vi "ExportDSAdata.vi"(8 "error in (no error)":errorcluster, 10 "Export Folder Path":path, 11 "Bode Plots":T1) -> (0 "error out":errorcluster)   [LabVIEW 2020, in "DynamicSignalAnalyzer.lvlib"]
doc: "Export DSA data to file"
uses:
  TypeDefs/BodePlot.ctl
  <vilib>/Utility/file.llb/Write Delimited Spreadsheet (DBL).vi
  DynamicSignalAnalyzer.lvlib
panel:
  in  "Pause Charts":bool
  # "For instructions on how to use the JKI State Machine Objects, examples and video tutorials, visit:\nhttp://jki.net/state-machine-objects/\n\nJKI State Machine Objects™\nhttp://jki.net/state-machine-objects/\nCopyright (C) 2005-2015, JKI <info@jki.net>\nALL RIGHTS RESERVED"
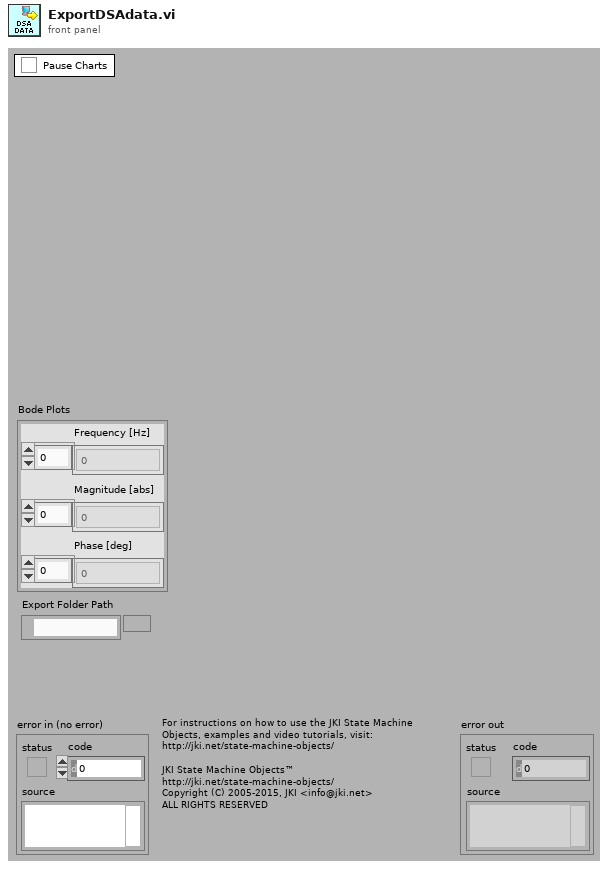
[diagram p1: front panel]
types:
  T1 = typedef "DynamicSignalAnalyzer.lvlib/BodePlot.ctl" = cluster{"Frequency [Hz]":dbl[], "Magnitude [abs]":dbl[], "Phase [deg]":dbl[]}
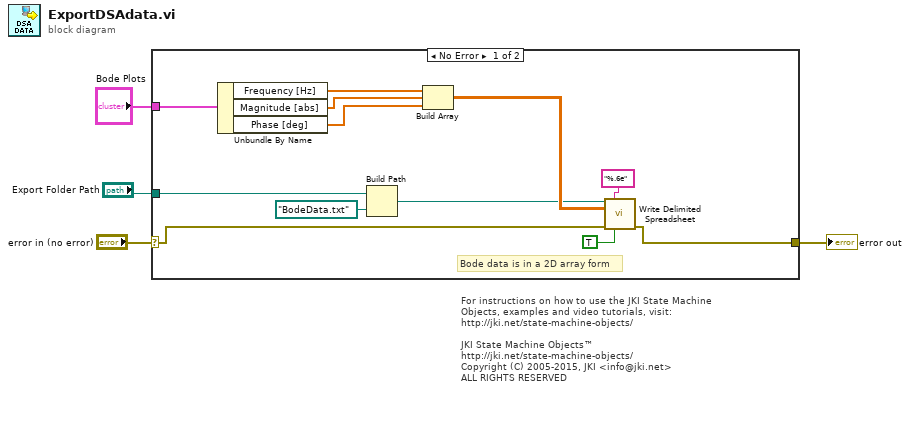
[diagram p0: block diagram]
diagram:
  # "For instructions on how to use the JKI State Machine Objects, examples and video tutorials, visit:\nhttp://jki.net/state-machine-objects/\n\nJKI State Machine Objects™\nhttp://jki.net/state-machine-objects/\nCopyright (C) 2005-2015, JKI <info@jki.net>\nALL RIGHTS RESERVED"
  n1 = case shown="No Error" "error in (no error)" {
    selector: "error in (no error)" -> [w6 w17]
    tunnel: [w5 w17] -> w4
    tunnel: "Export Folder Path" -> [w16 _]
    tunnel: "Bode Plots" -> [w12 _]
    frame No Error {
      # "Bode data is in a 2D array form"
      n2 = Unbundle By Name(w12) -> ("Frequency [Hz]"=w11:dbl[], "Magnitude [abs]"=w10:dbl[], "Phase [deg]"=w9:dbl[])
      n3 = Build Path(base path=w16, name or relative path=path "BodeData.txt") -> (appended path=w7:path)
      n4 = Build Array(w11, w10, w9) -> (w8:dbl[][])
      n5 = call-poly <vilib>:"Write Delimited Spreadsheet.vi"("file path (dialog if empty)"=w7, "format (%.3f)"="%.6e", "2D data"=w8, "error in (no error)"=w6, "transpose? (no:F)"=TRUE) -> ("error out"=w5:errorcluster)  [unwired: 9 in, 1 out]
    }
    frame Error {
    }
  }
  "error out" <- w4
